vi "Override To Nominal State.vi"(11 "Base Queue in":refnum<class "Base Queue.lvclass">) -> (3 "Base Queue out":refnum<class "Base Queue.lvclass">)   [LabVIEW 2021, in "jettl.lvlib" / "Base Queue.lvlib" / "Base Queue.lvclass"]
uses:
  Base Queue.lvclass
  State/Nominal State/Nominal State.lvclass
  C:/git/jettl/jettl/jettl/Base Queue/State/State/State.lvclass
  Base Queue.lvclass/Base Queue.ctl
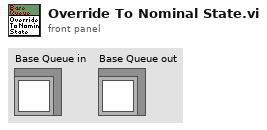
[diagram p1: front panel]
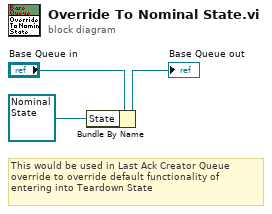
[diagram p0: block diagram]
diagram:
  # "This would be used in Last Ack Creator Queue override to override default functionality of entering into Teardown State"
  n1 = Bundle By Name(cluster="Base Queue in", "State"=refnum<class "Nominal State.lvclass"> refnum ("jettl.lvlib:Base Queue.lvlib:State.lvlib:Nominal State.lvclass")) -> (→"Base Queue out":refnum<class "Base Queue.lvclass">)
